vi "JAPCtiming4.vi"(8 "error in (no error)":errorcluster) -> (0 "error out":errorcluster)   [LabVIEW 2014]
uses:
  <userlib>/_RADE/RIO/JAPC/classes/JGet/openJAPCGet.vi
  <userlib>/_RADE/RIO/JAPC/classes/JGet/JAPCGet.vi
  <userlib>/_RADE/RIO/JAPC/classes/JGet/JGet.lvclass
panel:
  out "F-format string":string
  out "double precision float":dbl format="%#_11g"
  in  "stop":bool
  in  "URL":string
  out "data 2":dbl
  out "Instantaneous data":variant
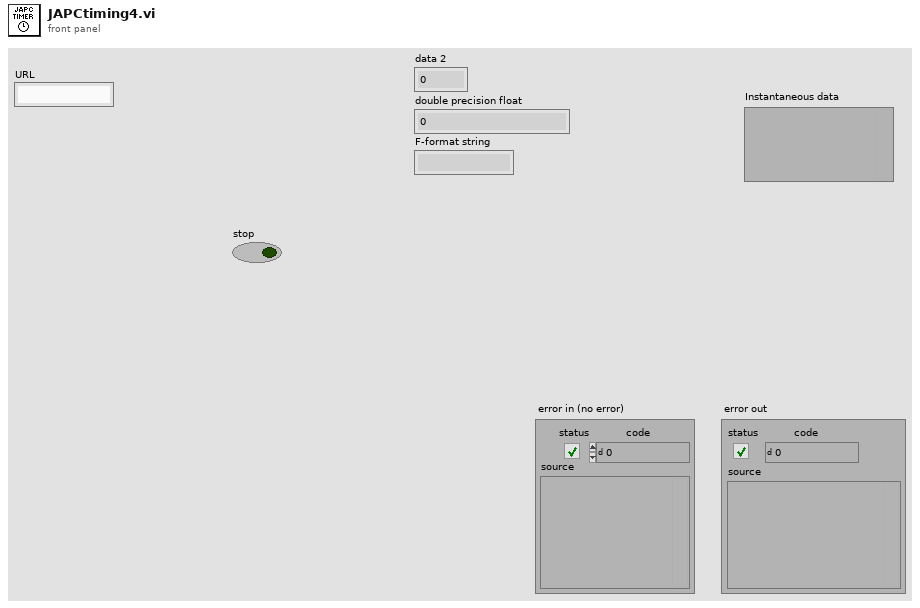
[diagram p1: front panel]
types:
  T1 = enum16{"open", "replace", "create", "open or create", "replace or create", "replace or create with confirmation"}
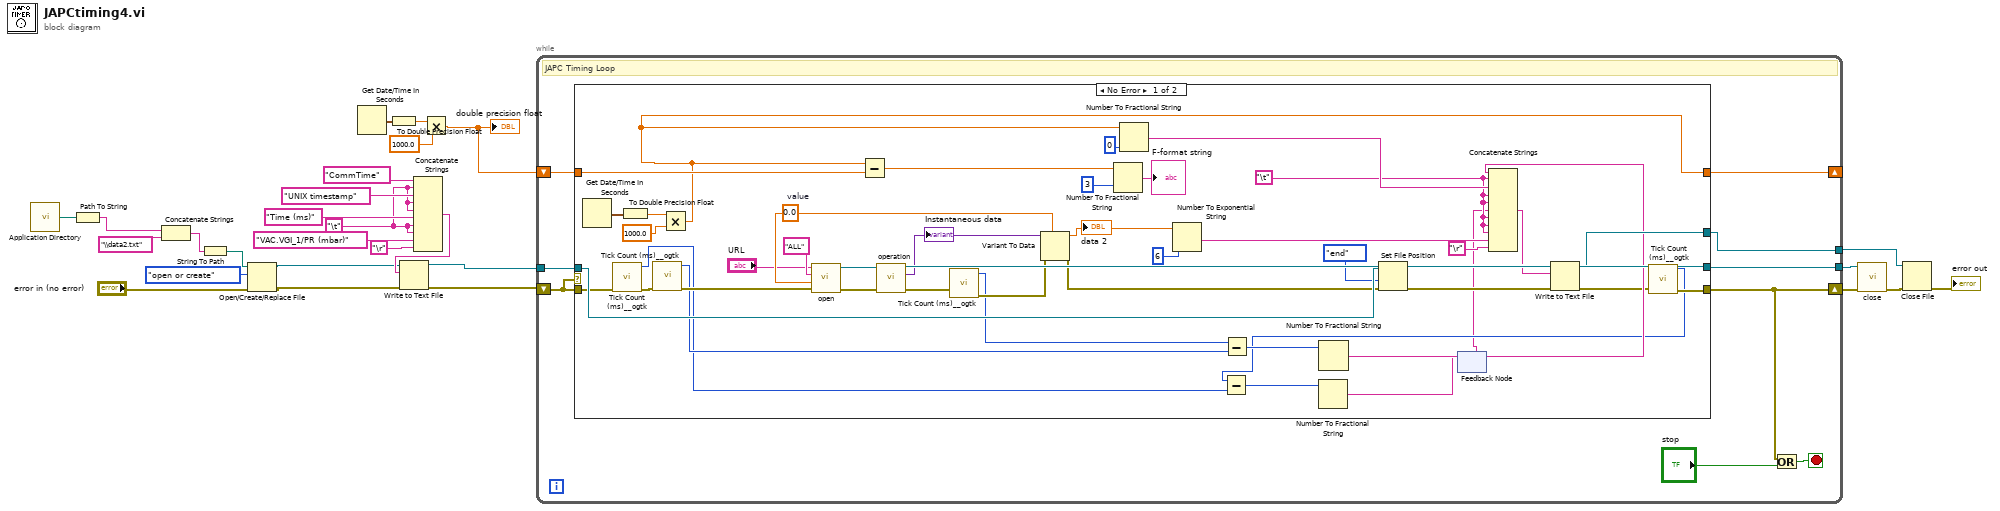
[diagram p0: block diagram]
diagram:
  w5 = "\t"
  n1 = call <vilib>:"Application Directory.vi"() -> ("Application Directory"=w20:path)
  n2 = Path To String(path=w20) -> (string=w19:string)
  n3 = Concatenate Strings(w19, "\\data2.txt" ("string")) -> (w16:string)
  n4 = String To Path(string=w16) -> (path=w17:path)
  n5 = Open/Create/Replace File(file path (use dialog)=w17, error in="error in (no error)", operation (0:open)=T1."open or create") -> (refnum out=w8:refnum<file>, error out=w9:errorcluster)  [unwired: 3 in, 1 out]
  n6 = Get Date/Time In Seconds() -> (seconds since 1Jan1904=w27:timestamp)
  n7 = To Double Precision Float(number=w27) -> (double precision float=w3:dbl)
  n8 = Concatenate Strings("CommTime" ("string"), w5, "UNIX timestamp" ("string"), w5, w5, "Time (ms)" ("string"), w5, w5, "VAC.VGI_1/PR (mbar)" ("string"), "\r") -> (w14:string)
  n9 = Write to Text File(file (use dialog)=w8, text=w14, error in=w9) -> (refnum out=w7:refnum<file>, error out=w4:errorcluster)  [unwired: 1 in, 1 out]
  n10 = Multiply(x=w3, y=1000.0) -> (x*y=w1:dbl)
  "double precision float" <- w1
  n11 = while {
    tunnel: [w36] -> w26
    shift-right: [w34] -> w25
    shift-left: w4 -> [w33]
    tunnel: [w32] -> w15
    tunnel: w7 -> [w30]
    shift-right: [w29] -> _
    shift-left: w1 -> [w28]
    stop <- w35 stop-if-true
    # "JAPC Timing Loop"
    n12 = case shown="No Error" w33 {
      tunnel: [w81 _] -> w36
      tunnel: [w44 w84] -> w34
      tunnel: w33 -> [w46 w84]
      tunnel: w30 -> [w73 w83]
      tunnel: [w74 w83] -> w32
      tunnel: [w47 w82] -> w29
      tunnel: w28 -> [w59 w82]
      frame No Error {
        w57 = "\t"
        w80 = 0.0  # value
        n13 = Get Date/Time In Seconds() -> (seconds since 1Jan1904=w50:timestamp)
        n14 = call <userlib>:"Tick Count (ms)__ogtk.vi"("error in (no error)"=w46) -> ("error out"=w45:errorcluster, "millisecond timer value"=w41:u32)  [unwired: 9 in]
        n15 = To Double Precision Float(number=w50) -> (double precision float=w49:dbl)
        n16 = call <userlib>:"Tick Count (ms)__ogtk.vi"("error in (no error)"=w45) -> ("error out"=w56:errorcluster, "millisecond timer value"=w52:u32)  [unwired: 9 in]
        n17 = Multiply(x=w49, y=1000.0) -> (x*y=w47:dbl)
        n18 = call-poly <userlib>:"open.vi"("error in (no error)"=w56, "Data type"=w80, "Cycle"="ALL", "URL"="URL") -> ("error out"=w79:errorcluster, "Object out"=w78:refnum<class "JGet.lvclass">)  [unwired: 6 in]
        n19 = Subtract(x=w47, y=w59) -> (x-y=w58:dbl)
        n20 = call-poly <userlib>:"operation.vi"("error in (no error)"=w79, "Object in"=w78) -> ("error out"=w55:errorcluster, "Data"=w76:variant, "Object out"=w81:refnum<class "JGet.lvclass">)  [unwired: 5 in, 2 out]
        "Instantaneous data" <- w76
        n21 = call <userlib>:"Tick Count (ms)__ogtk.vi"("error in (no error)"=w55) -> ("error out"=w54:errorcluster, "millisecond timer value"=w53:u32)  [unwired: 9 in]
        n22 = Variant To Data(error in=w54, type=w80, Variant=w76) -> (data=w63:dbl, error out=w71:errorcluster)
        "data 2" <- w63
        n23 = Number To Fractional String(number=w58, precision (6)=i16 3) -> (F-format string=→"F-format string":string)  [unwired: 2 in]
        n24 = Number To Fractional String(number=w47, precision (6)=i16 0) -> (F-format string=w67:string)  [unwired: 2 in]
        n25 = Number To Exponential String(number=w63, precision (6)=i16 6) -> (E-format string=w51:string)  [unwired: 2 in]
        n26 = Subtract(x=w53, y=w52) -> (x-y=w65:u32)
        n27 = Number To Fractional String(number=w65) -> (F-format string=w64:string)  [unwired: 3 in]
        n28 = Set File Position(refnum=w73, from (0:start)=enum16{"start", "end", "current"}."end", error in=w71) -> (refnum out=w69:refnum<file>, error out=w70:errorcluster)  [unwired: 1 in]
        n29 = feedback #1() -> (w38:string)  [unwired: 1 in]
        n30 = Concatenate Strings(w64, w57, w67, w57, w57, w38, w57, w57, w57, w51, "\r") -> (w66:string)
        n31 = Write to Text File(file (use dialog)=w69, text=w66, error in=w70) -> (refnum out=w74:refnum<file>, error out=w43:errorcluster)  [unwired: 1 in, 1 out]
        n32 = call <userlib>:"Tick Count (ms)__ogtk.vi"("error in (no error)"=w43) -> ("error out"=w44:errorcluster, "millisecond timer value"=w40:u32)  [unwired: 9 in]
        n33 = Subtract(x=w40, y=w41) -> (x-y=w42:u32)
        n34 = Number To Fractional String(number=w42) -> (F-format string=w39:string)  [unwired: 3 in]
        n35 = feedback-in #1(w39) -> ()
      }
      frame Error {
      }
    }
    n36 = Or(x=w34, y="stop") -> (x .or. y?=w35:bool)
  }
  n37 = call-dynamic "close.vi"("error in (no error)"=w25, "Object in"=w26) -> ("error out"=w24:errorcluster)  [unwired: 9 in]
  n38 = Close File(refnum=w15, error in=w24) -> (error out=→"error out":errorcluster)  [unwired: 1 out]
